vi "Init Bfr Tx - Create Buffer.vi"(8 "error in (no error)":errorcluster, 11 "Tx Loop Data in":T1 {"Data Buffer" format="%016x"}) -> (0 "error out":errorcluster, 3 "Tx Loop Data out":T1 {"Data Buffer" format="%016x"})   [LabVIEW 2016, in "UDP-Custom-Device Engine.lvlib"]
uses:
  UDP-Custom-Device Engine.lvlib
  Types/Engine - Buffered Tx Loop Data.ctl
  Shared/Types/Shared - Header Details.ctl
  Shared/Types/Shared - Buffered.PacketInfo.ctl
  <vilib>/NI/NIVS Inline Async API/_Data Access Engine/Data Access Engine/Types/ReadWrite.DVR.ctl
  <vilib>/NI/NIVS Inline Async API/_Data Access Engine/Access Type Classes/ReadWrite/ReadWrite.lvclass
  <vilib>/NI/NIVS Inline Async API/_Data Access Engine/Data Access Engine/Types/Read.DVR.ctl
  <vilib>/NI/NIVS Inline Async API/_Data Access Engine/Access Type Classes/Read/Read.lvclass
  <vilib>/NI/NIVS Inline Async API/_Data Access Engine/Data Access Engine/Types/Write.DVR.ctl
  <vilib>/NI/NIVS Inline Async API/_Data Access Engine/Access Type Classes/Write/Write.lvclass
  <vilib>/NI/NIVS Inline Async API/_Data Access Engine/Access Type Classes/Write/Write.lvclass/Write.ctl
  <vilib>/NI Veristand/VeriStand Data/Library/Pointer Operations/Pointer.Write (String).vi
  <vilib>/NI/NIVS Inline Async API/_Data Access Engine/Data Access Engine/Methods/Write.Data.vi
  <vilib>/NI/NIVS Inline Async API/_Data Access Engine/Access Type Classes/Write/Write.ProcessData.vi
  <vilib>/NI Veristand/VeriStand Data/Library/VeriStand Data.lvlib
  <vilib>/NI/NIVS Inline Async API/_Data Access Engine/Data Access Engine/Data Access Engine.lvclass
  Shared/UDP-Custom-Device Shared.lvlib
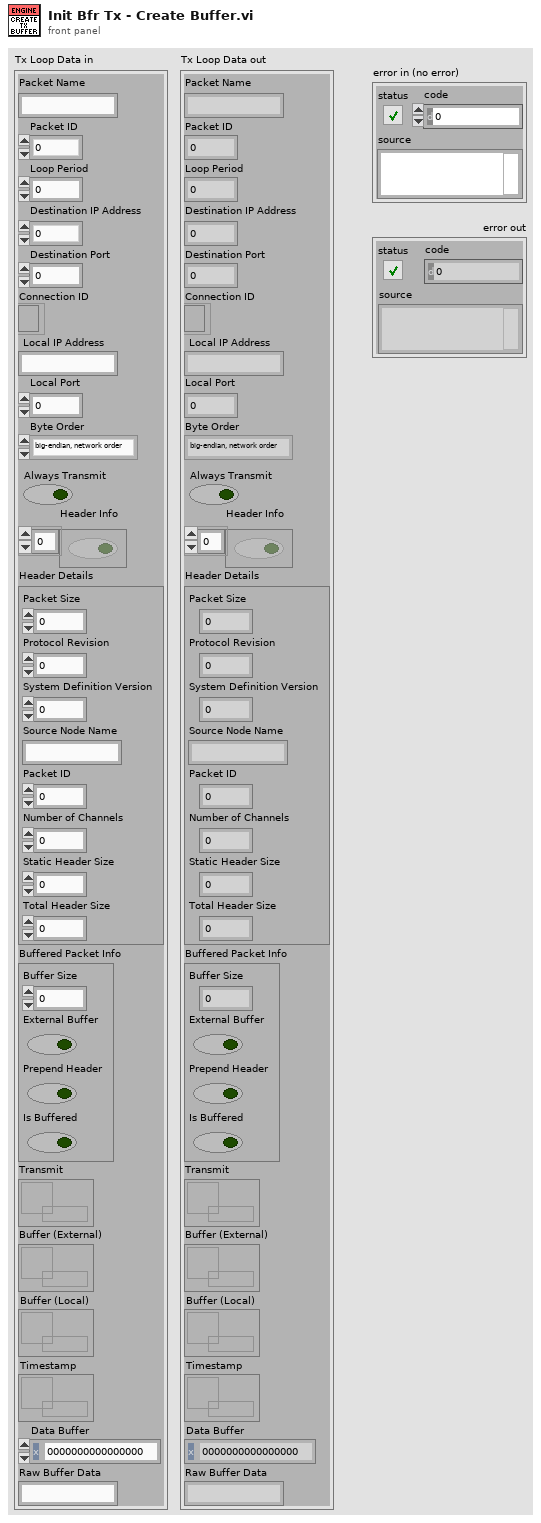
[diagram p1: front panel]
types:
  T1 = typedef "UDP-Custom-Device Engine.lvlib/Engine - Buffered Tx Loop Data.ctl" = cluster{"Packet Name":string, "Packet ID":i32, "Loop Period":u32, "Destination IP Address":u32, "Destination Port":u16, "Connection ID":refnum<k16>, "Local IP Address":string, "Local Port":i32, "Byte Order":enum16{"big-endian, network order", "native, host order", "little-endian"}, "Always Transmit":bool, "Header Info":bool[], "Header Details":T2, "Buffered Packet Info":T3, "Transmit":T4, "Buffer (External)":T5, "Buffer (Local)":T6, "Timestamp":T5, "Data Buffer":u64, "Raw Buffer Data":string}
  T2 = typedef "UDP-Custom-Device Shared.lvlib/Shared - Header Details.ctl" = cluster{"Packet Size":u16, "Protocol Revision":u8, "System Definition Version":u64, "Source Node Name":string, "Packet ID":u32, "Number of Channels":u32, "Static Header Size":u16, "Total Header Size":u16}
  T3 = typedef "UDP-Custom-Device Shared.lvlib/Shared - Buffered.PacketInfo.ctl" = cluster{"Buffer Size":i32, "External Buffer":bool, "Prepend Header":bool, "Is Buffered":bool}
  T4 = typedef "Data Access Engine.lvlib/Data Access Engine.lvclass/ReadWrite.DVR.ctl" = refnum<data-value>
  T5 = typedef "Data Access Engine.lvlib/Data Access Engine.lvclass/Read.DVR.ctl" = refnum<data-value>
  T6 = typedef "Data Access Engine.lvlib/Data Access Engine.lvclass/Write.DVR.ctl" = refnum<data-value>
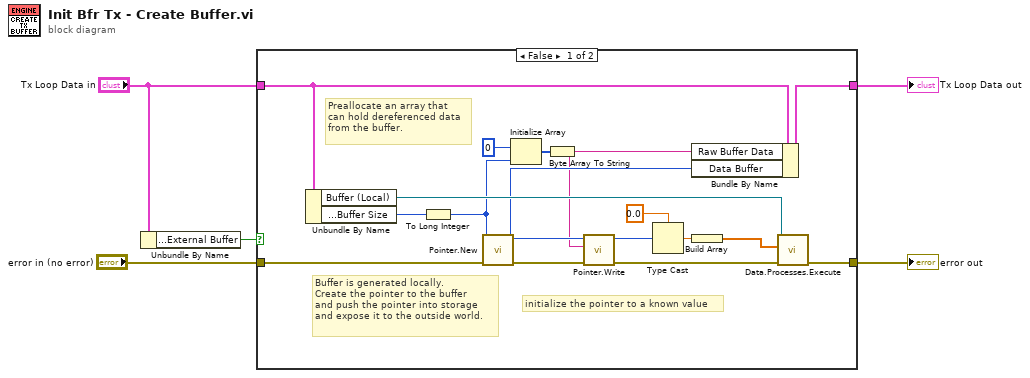
[diagram p0: block diagram]
diagram:
  n1 = Unbundle By Name("Tx Loop Data in") -> ("Buffered Packet Info.External Buffer"=w1:bool)
  n2 = case shown="False" w1 {
    tunnel: "error in (no error)" -> [w21 w23]
    tunnel: [w16 w23] -> w4
    tunnel: "Tx Loop Data in" -> [w20 w24]
    tunnel: [w19 w24] -> w3
    frame False {
      # "initialize the pointer to a known value"
      # "Preallocate an array that\ncan hold dereferenced data\nfrom the buffer."
      # "Buffer is generated locally.\nCreate the pointer to the buffer\nand push the pointer into storage\nand expose it to the outside world."
      n3 = Unbundle By Name(w20) -> ("Buffer (Local)"=w17:T6, "Buffered Packet Info.Buffer Size"=w22:i32)
      n4 = To Long Integer(number=w22) -> (32bit integer=w13:i32)
      n5 = call <vilib>:"Pointer.New.vi"("error in (no error)"=w21, "size in bytes"=w13) -> ("error out"=w8:errorcluster, "pointer"=w10:u64)  [unwired: 8 in]
      n6 = Initialize Array(u8 0, w13) -> (w11:u8[])
      n7 = Byte Array To String(unsigned byte array=w11) -> (string=w6:string)
      n8 = call-poly <vilib>:"Pointer.Write.vi"("error in (no error)"=w8, "string in"=w6, "pointer in"=w10) -> ("error out"=w7:errorcluster, "pointer out"=w9:u64)  [unwired: 6 in, 1 out]
      n9 = Type Cast(type=0.0, x=w9) -> (*(type *) &x=w15:dbl)
      n10 = Bundle By Name(cluster=w20, "Raw Buffer Data"=w6, "Data Buffer"=w10) -> (w19:T1)
      n11 = Build Array(w15) -> (w14:dbl[])
      n12 = call-poly <vilib>:"Data.Processes.Execute.vi"("error in (no error)"=w7, "Values"=w14, "Ref"=w17) -> ("error out"=w16:errorcluster)  [unwired: 8 in]
    }
    frame True {
    }
  }
  "Tx Loop Data out" <- w3
  "error out" <- w4
